vi "Read VSSParams.vi"(8 "error in (no error)":errorcluster, 11 "Parameters in":refnum<class "Parameters.lvclass">) -> (0 "error out":errorcluster, 2 "VSSParams":T1={"Robots ids"={"Goalie"=enum."0", "Attacker"=enum."1", "Defender"=enum."2"}}, 3 "Parameters out":refnum<class "Parameters.lvclass">)   [LabVIEW 2023, in "Parameters.lvclass"]
uses:
  Parameters.lvclass
  Parameters.lvclass/Parameters.ctl
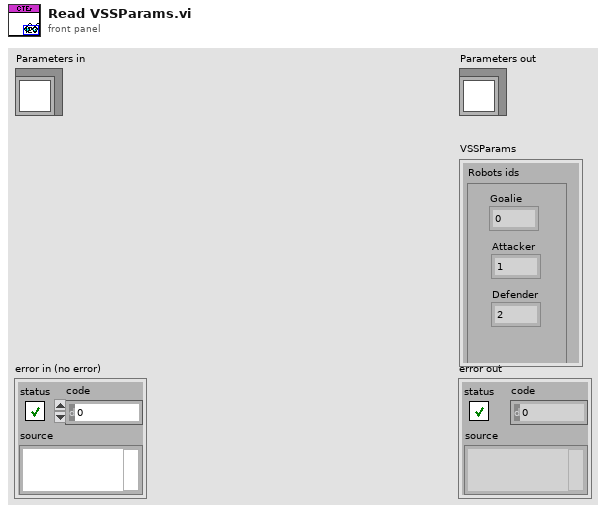
[diagram p1: front panel]
types:
  T1 = cluster{"Robots ids":cluster{"Goalie":enum16{"auto", "5", "4", "3", "2", "1", "0"}, "Attacker":enum16{"auto", "5", "4", "3", "2", "1", "0"}, "Defender":enum16{"auto", "5", "4", "3", "2", "1", "0"}}}
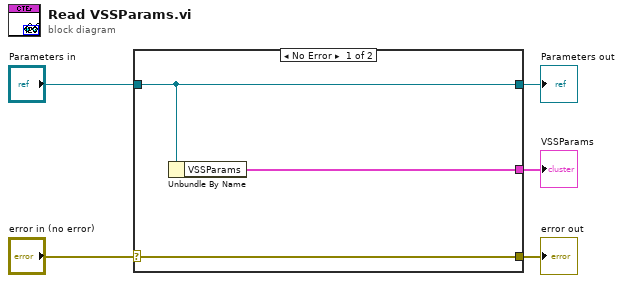
[diagram p0: block diagram]
diagram:
  n1 = case shown="No Error" "error in (no error)" {
    selector: "error in (no error)" -> [w8 w9]
    tunnel: [w8 w9] -> w4
    tunnel: [w7 w10] -> w2
    tunnel: "Parameters in" -> [w7 w10]
    tunnel: [w6 _] -> w1
    frame No Error {
      n2 = Unbundle By Name(w7) -> ("VSSParams"=w6:T1)
    }
    frame Error {
    }
  }
  "error out" <- w4
  "Parameters out" <- w2
  "VSSParams" <- w1
